vi "Roll station.vi"(0 "configuration file path":path caption="配置文件的路径", 1 "Roll station msic inf":T1) -> ()   [LabVIEW 2014]
uses:
  Ctl.xio/Roll station msic ctl.ctl
  SubVIS.xio/DataSocket/DataSocket_Tags.ctl
  Ctl.xio/part type.ctl
  <vilib>/Utility/file.llb/Read From Spreadsheet File (string).vi
  SubVIS.xio/Hopper car inf/Curing inf.vi
  SubVIS.xio/DataSocket/Write PLC Vars/Write Dbl Var in.vi
  SubVIS.xio/DataSocket/Write PLC Vars/Write Bool Var in.vi
panel:
  in  "SQL information":string
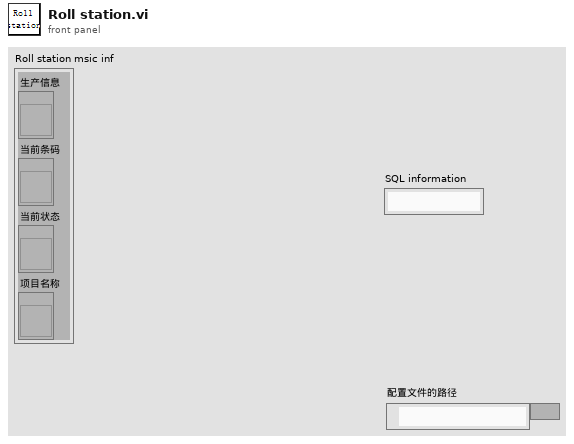
[diagram p1: front panel]
types:
  T1 = cluster{"生产信息":refnum<vi>, "当前条码":refnum<vi>, "当前状态":refnum<vi>, "项目名称":refnum<vi>}
  T2 = typedef "Roll station msic ctl.ctl" = cluster{"configuration file path":path, "DsOut":T3[], "Hopper car information":cluster{"Hopper car code":string, "Hopper car No":string, "plate No":string}, "pallet.produced number":i32, "SQL information":string, "Serial number":i32, "database path":path, "Roll station msic inf":cluster{"生产信息":refnum<vi>, "当前条码":refnum<vi>, "当前状态":refnum<vi>, "项目名称":refnum<vi>}, "part type":T4, "BarCode":string, "scanner resource name out":refnum<visa-resource-name>, "scanner coms or ip":string, "scanner ip ID":refnum<k5>, "curing timer":i32}
  T3 = typedef "DataSocket_Tags.ctl" = cluster{"Ds ID":refnum<k13>, "Tag":string}
  T4 = typedef "part type.ctl" = cluster{"项目号":string, "物料代码":string, "零件号":string, "供应商编码":string, "产线编码":string, "客户代码":string, "颜色代码":string, "托盘上限":i32, "加热温度":string, "加热时长":string, "EOL Stations":string}
  T5 = cluster{"Hopper car code":string, "Hopper car No":string, "plate No":string}
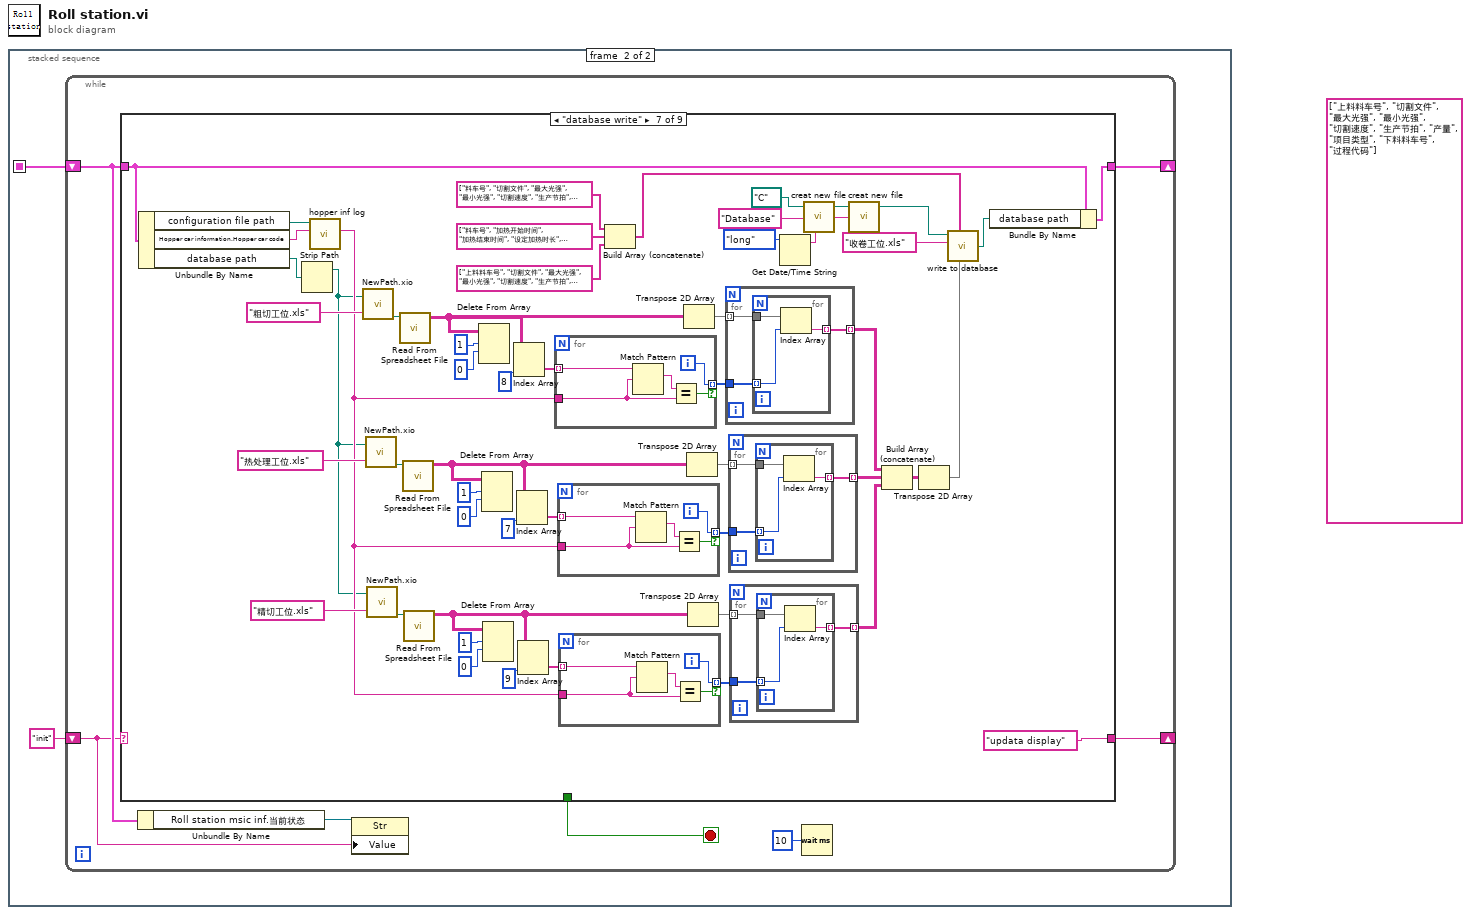
[diagram p0: block diagram]
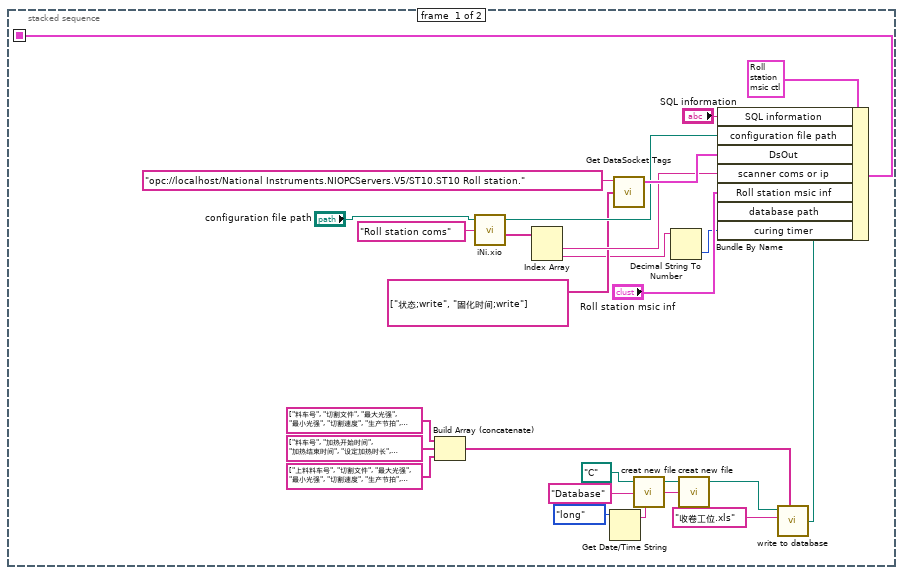
[diagram p2: hidden frame]
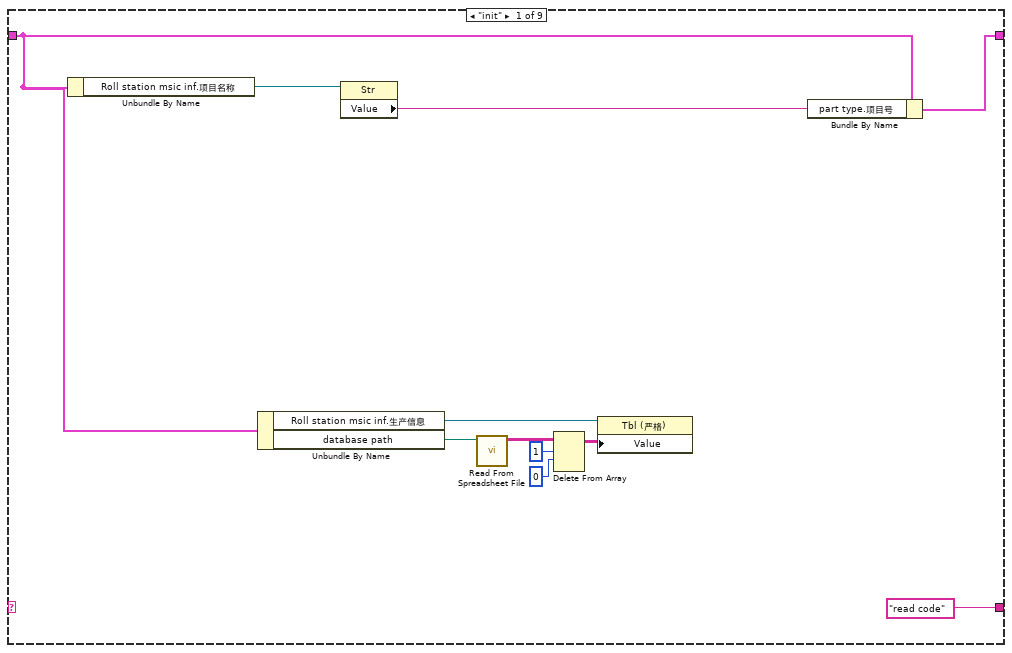
[diagram p3: hidden frame]
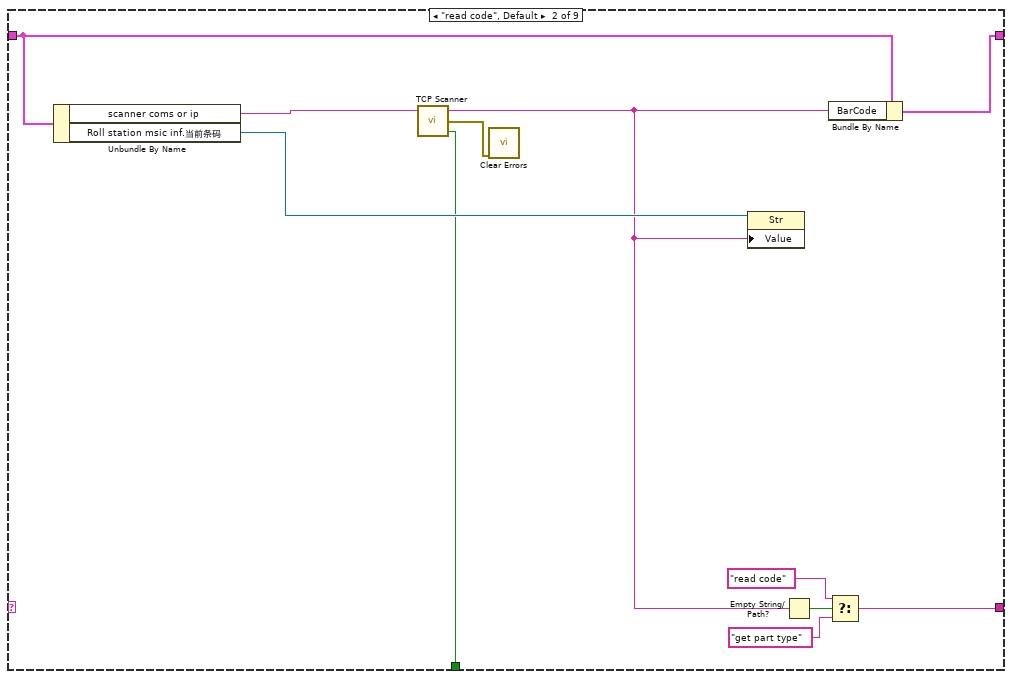
[diagram p4: hidden frame]
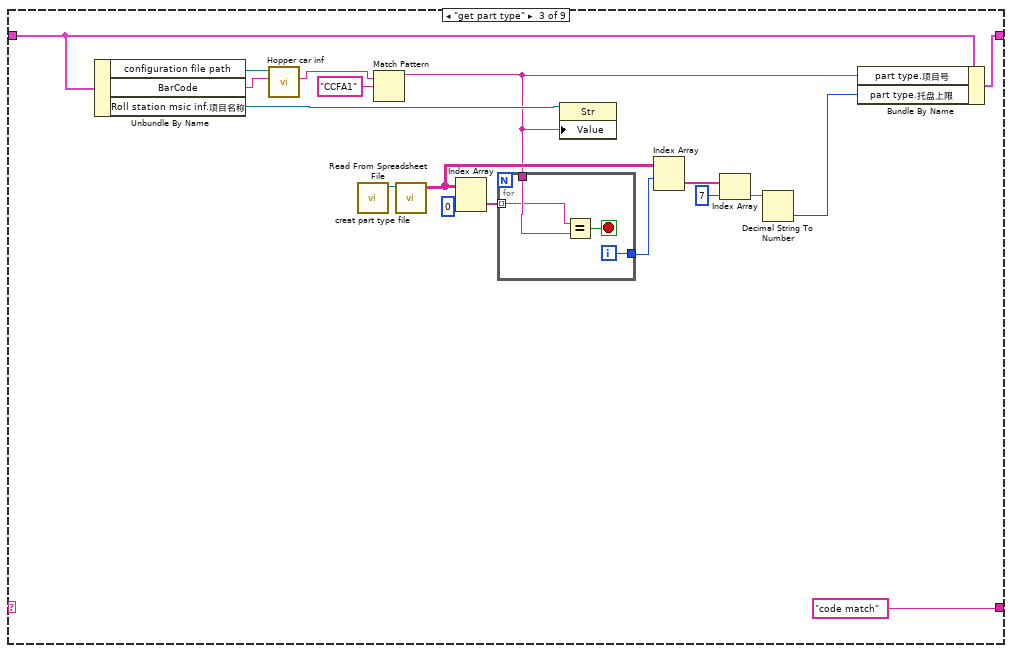
[diagram p5: hidden frame]
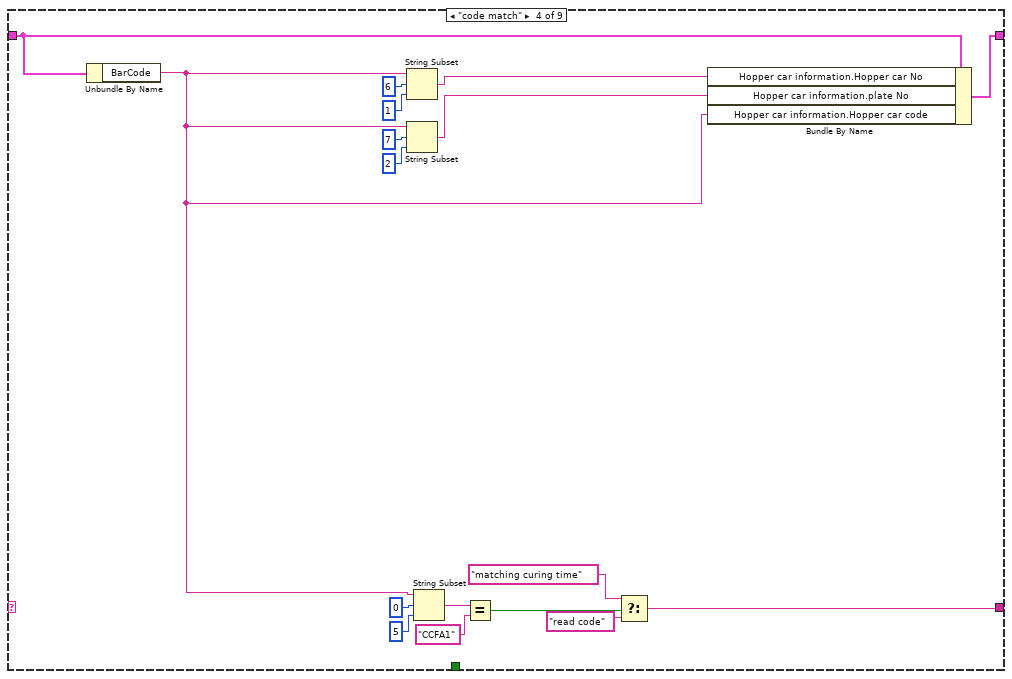
[diagram p6: hidden frame]
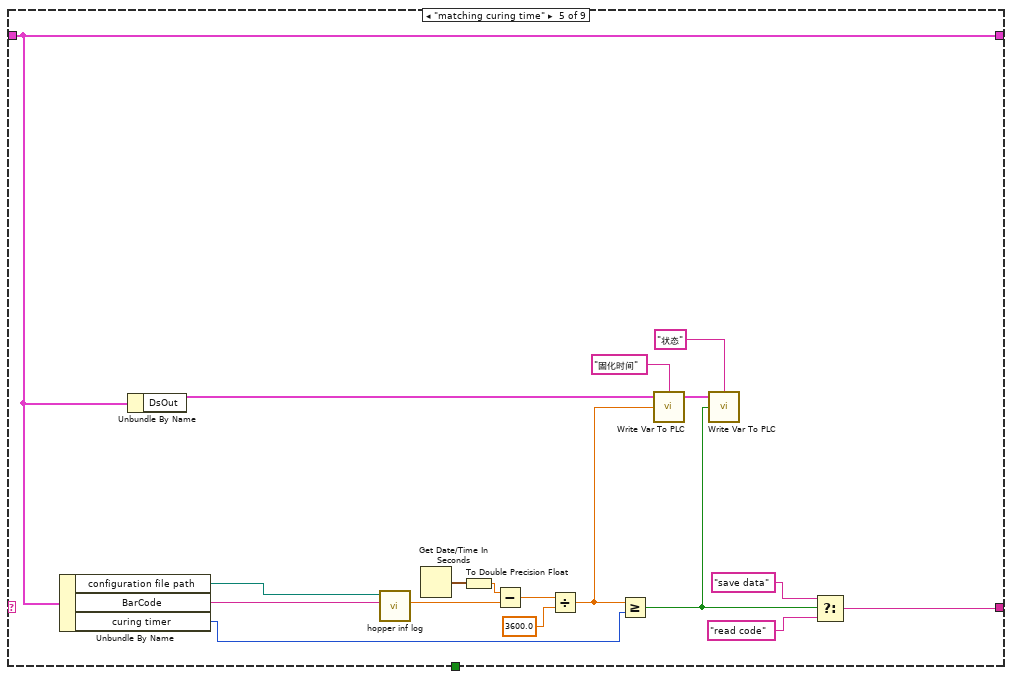
[diagram p7: hidden frame]
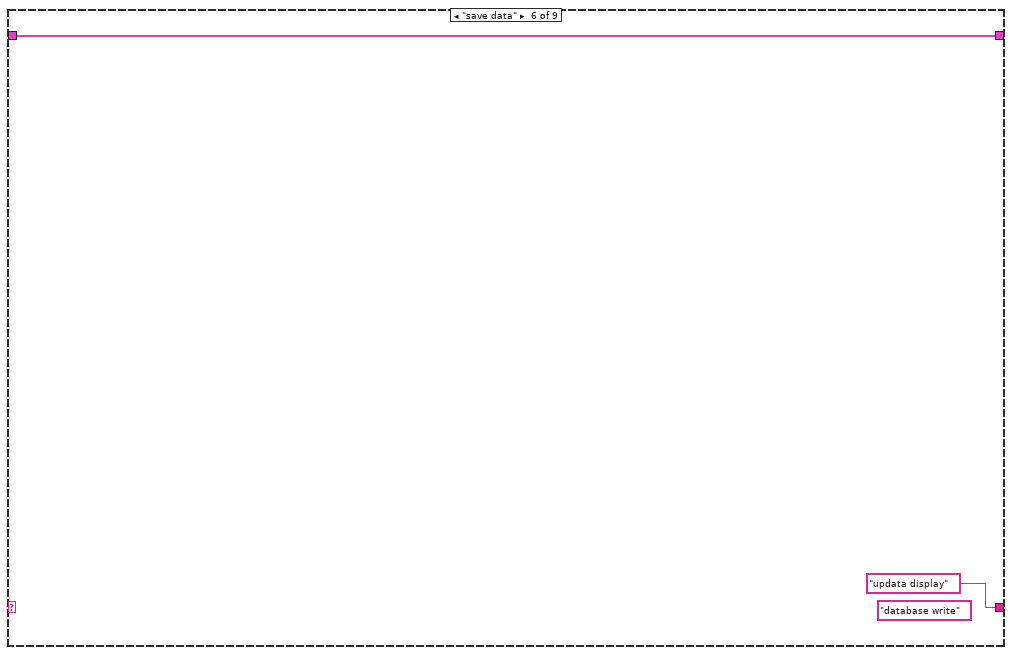
[diagram p8: hidden frame]
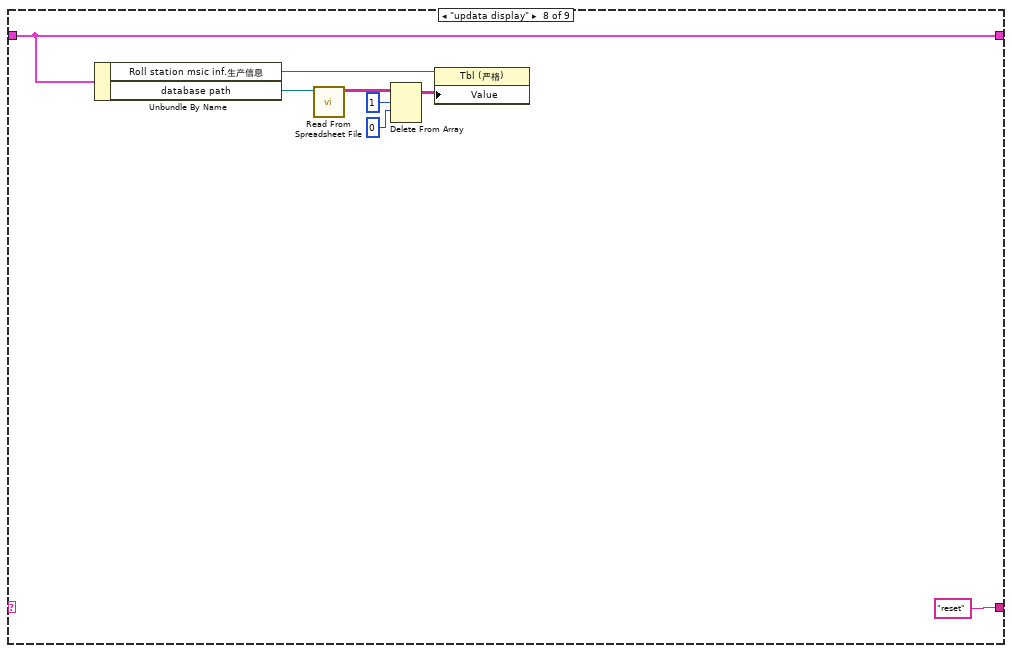
[diagram p9: hidden frame]
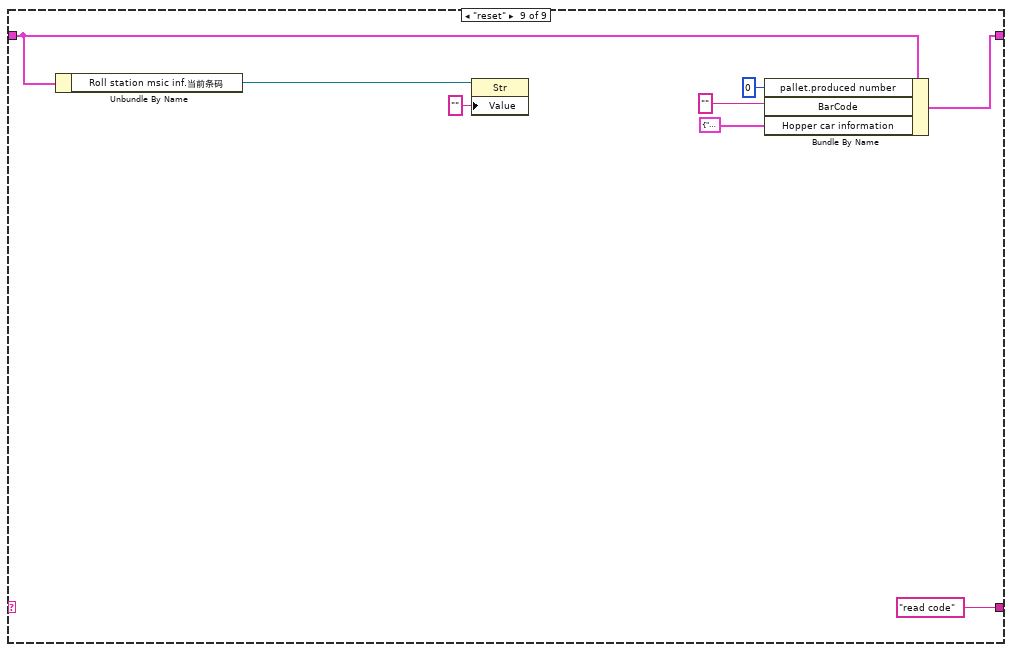
[diagram p10: hidden frame]
diagram:
  (unwired) string[] ["上料料车号", "切割文件", "最大光强", "最小光强", "切割速度", "生产节拍", "产量", "项目类型", "下料料车号", "过程代码"] ("Header")
  n1 = stacked-sequence {
    seq-local: [w17 _] -> [_ w27]
    frame #0 {
      n2 = Build Array (concatenate)(string[] ["料车号", "切割文件", "最大光强", "最小光强", "切割速度", "生产节拍", "产量", "项目类型", "过程条码"] ("Header"), string[] ["料车号", "加热开始时间", "加热结束时间", "设定加热时长", "实际加热时长", "设定加热温度", "项目类型", "过程代码"] ("Header"), string[] ["上料料车号", "切割文件", "最大光强", "最小光强", "切割速度", "生产节拍", "产量", "项目类型", "下料料车号", "过程代码"] ("Header")) -> (w4:string[])
      n3 = call "iNi.xio.vi"("configuration file path"="configuration file path", "Sections"="Roll station coms") -> ("configuration file path"=w25:path, "Values"=w23:string[])  [unwired: 1 in, 3 out]
      n4 = Index Array(array=w23) -> (element #1=w22:string, element #2=w1:string)  [unwired: 2 in]
      n5 = Get Date/Time String(date format (0)=enum16{"short", "long", "abbreviated"}."long" ("日期格式(0)")) -> (date string=w9:string)  [unwired: 2 in, 1 out]
      n6 = call "Get DataSocket Tags.vi"("All Tags"=string[] ["状态;write", "固化时间;write"], "URL"="opc://localhost/National Instruments.NIOPCServers.V5/ST10.ST10 Roll station.") -> ("DsOut"=w26:T3[])  [unwired: 3 in]
      n7 = call "creat new file.vi"("file name"="Database", "path"=path "C:/") -> ("created path"=w11:path)  [unwired: 1 in, 2 out]
      n8 = Decimal String To Number(string=w1) -> (number=w2:i32)  [unwired: 2 in, 1 out]
      n9 = call "creat new file.vi"("file name"=w9, "path"=w11) -> ("created path"=w10:path)  [unwired: 1 in, 2 out]
      n10 = call "write to database.vi"("Header"=w4, "file name"="收卷工位.xls", "path"=w10) -> ("new file path (Not A Path if cancelled)"=w3:path)  [unwired: 3 in]
      n11 = Bundle By Name(cluster=T2 {"configuration file path"=path "", "DsOut"=[], "Hopper car information"={"Hopper car code"="", "Hopper car No"="", "plate No"=""}, "pallet.produced number"=0, "SQL information"="", "Serial number"=0, "database path"=path "", "Roll station msic inf"={"生产信息"=refnum, "当前条码"=refnum, "当前状态"=refnum, "项目名称"=refnum}, "part type"={"项目号"="", "物料代码"="", "零件号"="", "供应商编码"="", "产线编码"="", "客户代码"="", "颜色代码"="", "托盘上限"=0, "加热温度"="", "加热时长"="", "EOL Stations"=""}, "BarCode"="", "scanner resource name out"="", "scanner coms or ip"="", "scanner ip ID"=refnum, "curing timer"=0} ("PDF Welding msic ctl"), "SQL information"="SQL information", "configuration file path"=w25, "DsOut"=w26, "scanner coms or ip"=w22, "Roll station msic inf"="Roll station msic inf", "database path"=w3, "curing timer"=w2) -> (w17:T2)
    }
    frame #1 {
      n12 = while {
        shift-right: [w35] -> _
        shift-left: w27 -> [w31]
        shift-right: [w34] -> _
        shift-left: "init" ("event") -> [w30]
        stop <- w29 stop-if-true
        n13 = case shown="\"database write\"" w30 {
          tunnel: w31 -> [w36 w55 w61 w82 w103 w115 w159 w206 w212]
          tunnel: [w46 w57 w75 w90 w103 w115 w163 w206 w216] -> w35
          tunnel: ["read code" w49 "code match" w89 w108 "updata display" ("f") "updata display" ("f") "reset" ("f") "read code" ("f")] -> w34
          tunnel: [_ w47 _ _ _ _ _ _ _] -> w29
          frame "init" {
            n14 = Unbundle By Name(w36) -> ("Roll station msic inf.项目名称"=w45:refnum<vi>)
            n15 = Unbundle By Name(w36) -> ("Roll station msic inf.生产信息"=w42:refnum<vi>, "database path"=w41:path)
            n16 = property class="Str"(reference=w45) -> ("Value"=w44:string)  [unwired: 1 in, 2 out]
            n17 = call-poly <vilib>:"Read From Spreadsheet File.vi"("file path (dialog if empty)"=w41) -> ("all rows"=w40:string[][])  [unwired: 6 in, 4 out]
            n18 = Delete From Array(array=w40, length=1 ("长度"), index (row)=0 ("索引 (行)")) -> (array with subset deleted=w37:string[][])  [unwired: 1 in, 1 out]
            n19 = property class="Tbl (严格)"(reference=w42, "Value"=w37) -> ()  [unwired: 1 in, 2 out]
            n20 = Bundle By Name(cluster=w36, "part type.项目号"=w44) -> (w46:T2)
          }
          frame "read code", Default {
            n21 = Unbundle By Name(w55) -> ("scanner coms or ip"=w54:string, "Roll station msic inf.当前条码"=w56:refnum<vi>)
            n22 = call "TCP Scanner.vi"("ip"=w54) -> ("status"=w47:bool, "错误输出"=w53:errorcluster, "Barcode"=w48:string)  [unwired: 2 in]
            n23 = call <vilib>:"Clear Errors.vi"("error in (no error)"=w53) -> ()  [unwired: 5 in, 2 out]
            n24 = property class="Str"(reference=w56, "Value"=w48) -> ()  [unwired: 1 in, 2 out]
            n25 = Empty String/Path?(string/path=w48) -> (empty?=w52:bool)
            n26 = Bundle By Name(cluster=w55, "BarCode"=w48) -> (w57:T2)
            n27 = Select(t="read code", s=w52, f="get part type") -> (s? t:f=w49:string)
          }
          frame "get part type" {
            n28 = Unbundle By Name(w61) -> ("configuration file path"=w65:path, "BarCode"=w64:string, "Roll station msic inf.项目名称"=w60:refnum<vi>)
            n29 = call "Hopper car inf.vi"("key"=w64, "path in"=w65) -> ("value out"=w63:string)  [unwired: 8 in, 1 out]
            n30 = call "creat part type file.vi"() -> ("new file path (Not A Path if cancelled)"=w66:path)  [unwired: 11 in]
            n31 = Match Pattern(string=w63, regular expression="CCFA1" ("正则表达式")) -> (before substring=w59:string)  [unwired: 1 in, 3 out]
            n32 = call-poly <vilib>:"Read From Spreadsheet File.vi"("file path (dialog if empty)"=w66) -> ("all rows"=w71:string[][])  [unwired: 6 in, 4 out]
            n33 = Index Array(array=w71, index (col)=0 ("禁用的索引 (列)")) -> (element=w73:string[])  [unwired: 1 in]
            n34 = for {
              tunnel: w73 -> [w76] mode=indexing
              tunnel: [w78] -> w70
              tunnel: w59 -> [w77]
              i -> [w78]
              stop <- w79 stop-if-true
              n35 = Equal?(x=w76, y=w77) -> (x = y?=w79:bool)
            }
            n36 = property class="Str"(reference=w60, "Value"=w59) -> ()  [unwired: 1 in, 2 out]
            n37 = Index Array(array=w71, index (row)=w70) -> (element=w69:string[])  [unwired: 1 in]
            n38 = Index Array(array=w69, index=7 ("索引")) -> (element=w68:string)
            n39 = Decimal String To Number(string=w68) -> (number=w67:i32)  [unwired: 2 in, 1 out]
            n40 = Bundle By Name(cluster=w61, "part type.项目号"=w59, "part type.托盘上限"=w67) -> (w75:T2)
          }
          frame "code match" {
            n41 = Unbundle By Name(w82) -> ("BarCode"=w81:string)
            n42 = String Subset(string=w81, offset (0)=6 ("偏移量(0)"), length (rest)=1 ("长度（剩余）")) -> (substring=w84:string)
            n43 = String Subset(string=w81, offset (0)=7 ("偏移量(0)"), length (rest)=2 ("长度（剩余）")) -> (substring=w85:string)
            n44 = String Subset(string=w81, offset (0)=0 ("偏移量(0)"), length (rest)=5 ("长度（剩余）")) -> (substring=w86:string)
            n45 = Equal?(x=w86, y="CCFA1") -> (x = y?=w80:bool)
            n46 = Select(t="matching curing time" ("event"), s=w80, f="read code" ("event")) -> (s? t:f=w89:string)
            n47 = Bundle By Name(cluster=w82, "Hopper car information.Hopper car No"=w84, "Hopper car information.plate No"=w85, "Hopper car information.Hopper car code"=w81) -> (w90:T2)
          }
          frame "matching curing time" {
            n48 = Unbundle By Name(w103) -> ("configuration file path"=w114:path, "BarCode"=w113:string, "curing timer"=w106:i32)
            n49 = Unbundle By Name(w103) -> ("DsOut"=w102:T3[])
            n50 = call-poly "hopper inf log.vi"("key"=w113, "path in"=w114) -> ("value out"=w104:dbl)  [unwired: 8 in, 1 out]
            n51 = Get Date/Time In Seconds() -> (seconds since 1Jan1904=w112:timestamp)
            n52 = To Double Precision Float(number=w112) -> (double precision float=w105:dbl)
            n53 = Subtract(x=w105, y=w104) -> (x-y=w111:dbl)
            n54 = Divide(x=w111, y=3600.0) -> (x/y=w98:dbl)
            n55 = Greater Or Equal?(x=w98, y=w106) -> (x >= y?=w97:bool)
            n56 = call-poly "Write Var To PLC.vi"("Tag IN"="固化时间", "Dbl Var in"=w98, "Ds PLCTags IN"=w102) -> ("Ds PLCTags OUT"=w100:T3[])  [unwired: 1 in, 1 out]
            n57 = call-poly "Write Var To PLC.vi"("Tag IN"="状态", "Bool Var in"=w97, "Ds PLCTags IN"=w100) -> ()  [unwired: 1 in, 2 out]
            n58 = Select(t="save data" ("event"), s=w97, f="read code") -> (s? t:f=w108:string)
          }
          frame "save data" {
            (unwired) "database write" ("f")
          }
          frame "database write" {
            n59 = Unbundle By Name(w159) -> ("configuration file path"=w158:path, "Hopper car information.Hopper car code"=w156:string, "database path"=w118:path)
            n60 = Strip Path(path=w118) -> (stripped path=w117:path)  [unwired: 1 out]
            n61 = call-poly "hopper inf log.vi"("key"=w156, "path in"=w158) -> ("value out"=w128:string)  [unwired: 8 in, 1 out]
            n62 = call "NewPath.xio.vi"("Append path"="粗切工位.xls", "Basic path"=w117) -> ("New path"=w148:path)
            n63 = call "NewPath.xio.vi"("Append path"="热处理工位.xls", "Basic path"=w117) -> ("New path"=w145:path)
            n64 = call "NewPath.xio.vi"("Append path"="精切工位.xls", "Basic path"=w117) -> ("New path"=w130:path)
            n65 = call-poly <vilib>:"Read From Spreadsheet File.vi"("file path (dialog if empty)"=w148) -> ("all rows"=w149:string[][])  [unwired: 6 in, 4 out]
            n66 = call-poly <vilib>:"Read From Spreadsheet File.vi"("file path (dialog if empty)"=w145) -> ("all rows"=w144:string[][])  [unwired: 6 in, 4 out]
            n67 = call-poly <vilib>:"Read From Spreadsheet File.vi"("file path (dialog if empty)"=w130) -> ("all rows"=w131:string[][])  [unwired: 6 in, 4 out]
            n68 = Delete From Array(array=w149, length=1 ("长度"), index (row)=0 ("索引 (行)")) -> ()  [unwired: 1 in, 2 out]
            n69 = Delete From Array(array=w144, length=1 ("长度"), index (row)=0 ("索引 (行)")) -> ()  [unwired: 1 in, 2 out]
            n70 = Delete From Array(array=w131, length=1 ("长度"), index (row)=0 ("索引 (行)")) -> ()  [unwired: 1 in, 2 out]
            n71 = Index Array(array=w149, index (col)=8 ("禁用的索引 (列)")) -> (element=w153:string[])  [unwired: 1 in]
            n72 = Index Array(array=w144, index (col)=7 ("禁用的索引 (列)")) -> (element=w140:string[])  [unwired: 1 in]
            n73 = Index Array(array=w131, index (col)=9 ("禁用的索引 (列)")) -> (element=w135:string[])  [unwired: 1 in]
            n74 = for {
              tunnel: w153 -> [w195] mode=indexing
              tunnel: [w193] -> w152 mode=indexing if=w192
              tunnel: w128 -> [w191]
              i -> [w193]
              n75 = Match Pattern(string=w195, regular expression=w191) -> (match substring=w194:string)  [unwired: 1 in, 3 out]
              n76 = Equal?(x=w194, y=w191) -> (x = y?=w192:bool)
            }
            n77 = for {
              tunnel: w140 -> [w184] mode=indexing
              tunnel: [w182] -> w141 mode=indexing if=w181
              tunnel: w128 -> [w180]
              i -> [w182]
              n78 = Match Pattern(string=w184, regular expression=w180) -> (match substring=w183:string)  [unwired: 1 in, 3 out]
              n79 = Equal?(x=w183, y=w180) -> (x = y?=w181:bool)
            }
            n80 = for {
              tunnel: w135 -> [w173] mode=indexing
              tunnel: [w171] -> w134 mode=indexing if=w170
              tunnel: w128 -> [w169]
              i -> [w171]
              n81 = Match Pattern(string=w173, regular expression=w169) -> (match substring=w172:string)  [unwired: 1 in, 3 out]
              n82 = Equal?(x=w172, y=w169) -> (x = y?=w170:bool)
            }
            n83 = Build Array (concatenate)(string[] ["料车号", "切割文件", "最大光强", "最小光强", "切割速度", "生产节拍", "产量", "项目类型", "过程条码"] ("Header"), string[] ["料车号", "加热开始时间", "加热结束时间", "设定加热时长", "实际加热时长", "设定加热温度", "项目类型", "过程代码"] ("Header"), string[] ["上料料车号", "切割文件", "最大光强", "最小光强", "切割速度", "生产节拍", "产量", "项目类型", "下料料车号", "过程代码"] ("Header")) -> (w119:string[])
            n84 = Transpose 2D Array(2D array=w149) -> (transposed array=w150:string[][])
            n85 = Transpose 2D Array(2D array=w144) -> (transposed array=w143:string[][])
            n86 = Transpose 2D Array(2D array=w131) -> (transposed array=w132:string[][])
            n87 = for {
              tunnel: w150 -> [w198] mode=indexing
              tunnel: w152 -> [w197]
              tunnel: [w196] -> w126 mode=indexing
              n88 = for {
                tunnel: w198 -> [w201]
                tunnel: w197 -> [w200] mode=indexing
                tunnel: [w199] -> w196 mode=indexing
                n89 = Index Array(array=w201, index=w200) -> (element=w199:string)
              }
            }
            n90 = for {
              tunnel: w143 -> [w187] mode=indexing
              tunnel: w141 -> [w186]
              tunnel: [w185] -> w127 mode=indexing
              n91 = for {
                tunnel: w187 -> [w190]
                tunnel: w186 -> [w189] mode=indexing
                tunnel: [w188] -> w185 mode=indexing
                n92 = Index Array(array=w190, index=w189) -> (element=w188:string)
              }
            }
            n93 = for {
              tunnel: w132 -> [w176] mode=indexing
              tunnel: w134 -> [w175]
              tunnel: [w174] -> w125 mode=indexing
              n94 = for {
                tunnel: w176 -> [w179]
                tunnel: w175 -> [w178] mode=indexing
                tunnel: [w177] -> w174 mode=indexing
                n95 = Index Array(array=w179, index=w178) -> (element=w177:string)
              }
            }
            n96 = Get Date/Time String(date format (0)=enum16{"short", "long", "abbreviated"}."long" ("日期格式(0)")) -> (date string=w160:string)  [unwired: 2 in, 1 out]
            n97 = call "creat new file.vi"("file name"="Database", "path"=path "C:/") -> ("created path"=w162:path)  [unwired: 1 in, 2 out]
            n98 = call "creat new file.vi"("file name"=w160, "path"=w162) -> ("created path"=w161:path)  [unwired: 1 in, 2 out]
            n99 = Build Array (concatenate)(w126, w127, w125) -> (w124:string[][])
            n100 = Transpose 2D Array(2D array=w124) -> (transposed array=w123:string[][])
            n101 = call "write to database.vi"("2D data"=w123, "Header"=w119, "file name"="收卷工位.xls", "path"=w161) -> ("new file path (Not A Path if cancelled)"=w164:path)  [unwired: 2 in]
            n102 = Bundle By Name(cluster=w159, "database path"=w164) -> (w163:T2)
          }
          frame "updata display" {
            n103 = Unbundle By Name(w206) -> ("Roll station msic inf.生产信息"=w208:refnum<vi>, "database path"=w207:path)
            n104 = call-poly <vilib>:"Read From Spreadsheet File.vi"("file path (dialog if empty)"=w207) -> ("all rows"=w205:string[][])  [unwired: 6 in, 4 out]
            n105 = Delete From Array(array=w205, length=1 ("长度"), index (row)=0 ("索引 (行)")) -> (array with subset deleted=w202:string[][])  [unwired: 1 in, 1 out]
            n106 = property class="Tbl (严格)"(reference=w208, "Value"=w202) -> ()  [unwired: 1 in, 2 out]
          }
          frame "reset" {
            n107 = Unbundle By Name(w212) -> ("Roll station msic inf.当前条码"=w211:refnum<vi>)
            n108 = property class="Str"(reference=w211, "Value"="" ("值")) -> ()  [unwired: 1 in, 2 out]
            n109 = Bundle By Name(cluster=w212, "pallet.produced number"=0, "BarCode"="", "Hopper car information"=T5 {"Hopper car code"="", "Hopper car No"="", "plate No"=""}) -> (w216:T2)
          }
        }
        n110 = Unbundle By Name(w31) -> ("Roll station msic inf.当前状态"=w32:refnum<vi>)
        n111 = property class="Str"(reference=w32, "Value"=w30) -> ()  [unwired: 1 in, 2 out]
        n112 = Wait (ms)(milliseconds to wait=u32 10 ("等待时间（毫秒）")) -> ()  [unwired: 1 out]
      }
    }
  }
